vi "fgv_Patch viewer internal register.vi"(9 "Function":T3, 11 "Registered setup":T1) -> (3 "Registered setup":T1)   [LabVIEW 2017]
uses:
  Typedefs/Read Write Enum.ctl
  Typedefs/Patch viewer internal cluster.ctl
  <vilib>/vision/Image Controls.llb/IMAQ Image.ctl
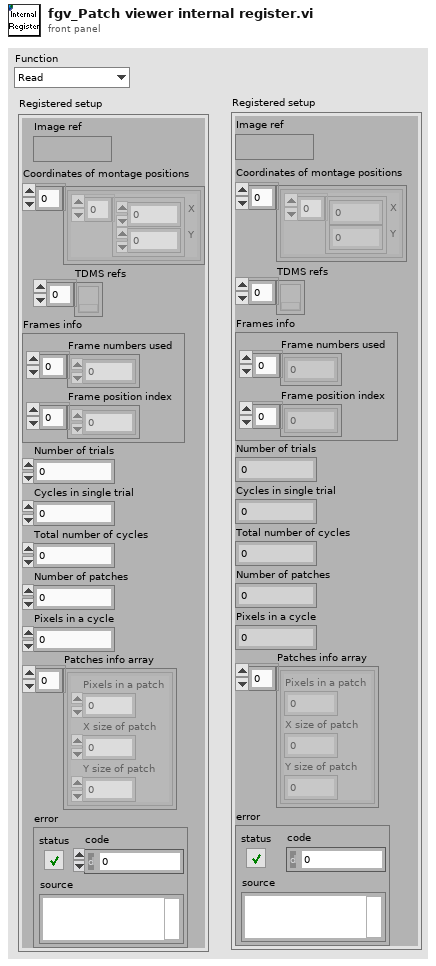
[diagram p1: front panel]
types:
  T1 = typedef "Patch viewer internal cluster.ctl" = cluster{"Image ref":T2, "Coordinates of montage positions":cluster{"X\n\nY":i32[]}[], "TDMS refs":refnum<k34>[], "Frames info":cluster{"Frame numbers used":i32[], "Frame position index":i32[]}, "Number of trials":i32, "Cycles in single trial":i32, "Total number of cycles":i32, "Number of patches":i32, "Pixels in a cycle":i32, "Patches info array":cluster{"Pixels in a patch":i32, "X size of patch":i32, "Y size of patch":i32}[], "error":errorcluster}
  T2 = typedef "IMAQ Image.ctl" = refnum<image>
  T3 = typedef "Read Write Enum.ctl" = enum16{"Read", "Write"}
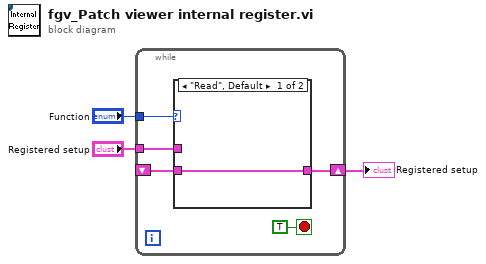
[diagram p0: block diagram]
diagram:
  n1 = while {
    tunnel: "Function" -> [w7]
    tunnel: "Registered setup" -> [w6]
    shift-right: [w5] -> w1
    shift-left: _ -> [w4]
    stop <- TRUE stop-if-true
    n2 = case shown="\"Read\", Default" w7 {
      tunnel: w6 -> [_ w10]
      tunnel: [w9 w10] -> w5
      tunnel: w4 -> [w9 _]
      frame "Read", Default {
      }
      frame "Write" {
      }
    }
  }
  "Registered setup" <- w1
